vi "PhotonMultiTargetPNPResult_MAX_IDS.vi"() -> (3 "MAX_IDS":i32=32)   [LabVIEW 2019, in "PhotonVisionLib.lvlib"]
uses:
  PhotonVisionLib.lvlib
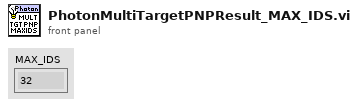
[diagram p1: front panel]
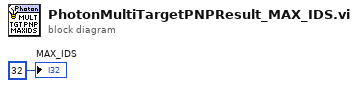
[diagram p0: block diagram]
diagram:
  "MAX_IDS" <- 32 ("MAX_IDS")
